vi "Results.vi"(8 "error in (no error)":errorcluster, 11 "User Interface in":refnum<class "User Interface.lvclass">) -> (0 "error out":errorcluster, 3 "User Interface out":refnum<class "User Interface.lvclass">)   [LabVIEW 2020, in "User Interface.lvlib" / "User Interface.lvclass"]
uses:
  User Interface.lvclass
  User Interface.lvclass/User Interface.ctl
  <vilib>/drjdpowell/SQLite Library/SQL Connection/Open (path).vi
  <vilib>/drjdpowell/SQLite Library/SQL Connection/Open (string).vi
  <vilib>/AdvancedString/Path To Command Line String.vi
  <vilib>/drjdpowell/SQLite Library/SQL Connection/Execute SQL.vi
  <vilib>/drjdpowell/SQLite Library/SQL Connection/Connection.lvclass
  <vilib>/drjdpowell/SQLite Library/SQLite.lvlib
panel:
  in  "WasCar Database":i32(listbox)
  in  "Exit":bool
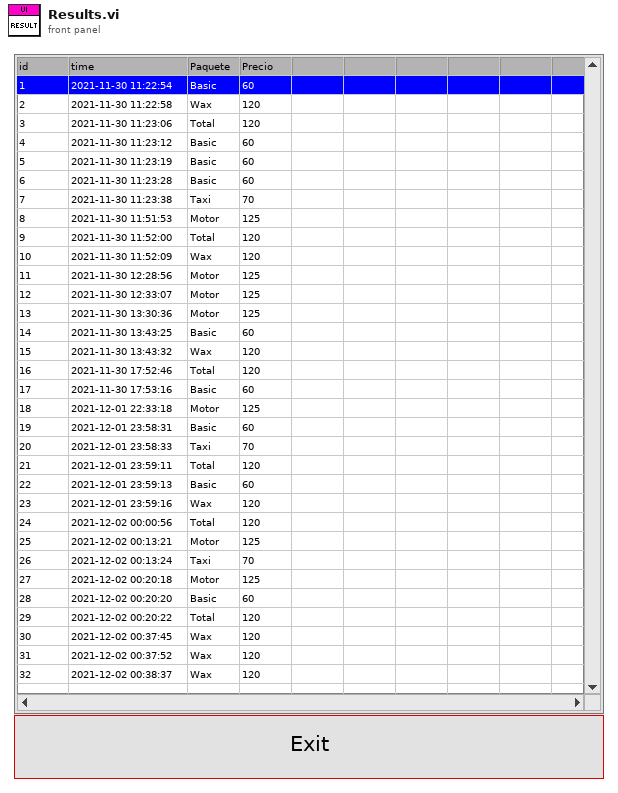
[diagram p1: front panel]
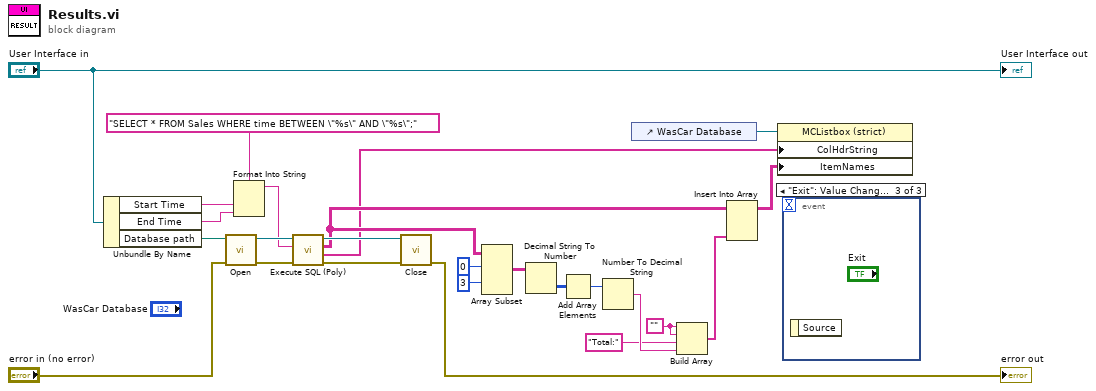
[diagram p0: block diagram]
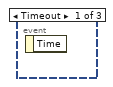
[diagram p2: hidden frame]
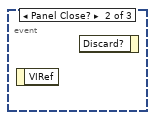
[diagram p3: hidden frame]
diagram:
  w4 = ""
  n1 = Unbundle By Name("User Interface in") -> ("Start Time"=w23:string, "End Time"=w22:string, "Database path"=w21:path)
  n2 = call-poly <vilib>:"Open.vi"("error in (no error)"="error in (no error)", "db file"=w21) -> ("error out"=w19:errorcluster, "SQLite Connection"=w18:refnum<class "Connection.lvclass">)  [unwired: 8 in]
  n3 = Format Into String(format string="SELECT * FROM Sales WHERE time BETWEEN \"%s\" AND \"%s\";" ("SQL"), w23, w22) -> (resulting string=w17:string)  [unwired: 2 in, 1 out]
  n4 = call-poly <vilib>:"Execute SQL (Poly).vi"("error in (no error)"=w19, "SQL"=w17, "SQLite Connection in"=w18) -> ("error out"=w16:errorcluster, "Column Names"=w2:string[], "Result Set"=w12:string[][], "SQLite Connection"=w14:refnum<class "Connection.lvclass">)  [unwired: 5 in]
  n5 = call-dynamic "Close.vi"("error in (no error)"=w16, "SQLite Connection in"=w14) -> ("error out"=→"error out":errorcluster)  [unwired: 9 in]
  n6 = Array Subset(array=w12, index (row)=0 ("index"), index (col)=3 ("index")) -> (w9:string[][])  [unwired: 2 in]
  n7 = Decimal String To Number(string=w9) -> (number=w8:i32[][])  [unwired: 2 in, 1 out]
  n8 = Add Array Elements(numeric array=w8) -> (sum=w7:i32)
  n9 = Number To Decimal String(number=w7) -> (decimal integer string=w6:string)  [unwired: 1 in]
  n10 = control-ref of="WasCar Database"() -> (w13:refnum<vi>)
  n11 = Build Array(w4, w4, "Total:" ("element"), w6) -> (w3:string[])
  n12 = Insert Into Array(array=w12, new element=w3) -> (w1:string[][])  [unwired: 2 in]
  n13 = property class="MCListbox (strict)"(reference=w13, "ColHdrString"=w2, "ItemNames"=w1) -> ()  [unwired: 1 in, 2 out]
  n14 = event shown="[2] \"Exit\": Value Change" {
    selector: _ -> [_ _ _]
    dyn-events: _ -> [_ _ _]
    timeout: _ -> [_ _ _]
    event Timeout {
      n15 = event-data() -> ()  [unwired: 1 in, 1 out]
    }
    event Panel Close? {
      n16 = event-data() -> ()  [unwired: 1 in, 1 out]
      n17 = event-data() -> ()  [unwired: 2 in, 1 out]
    }
    event "Exit": Value Change {
      n18 = event-data() -> ()  [unwired: 1 in, 1 out]
    }
  }
  "User Interface out" <- "User Interface in"
